vi "Write.vi"(8 "error in (no error)":errorcluster, 10 "Boolean":bool, 11 "Boolean Constant in":refnum<class "Boolean.lvclass">) -> (0 "error out":errorcluster, 3 "Boolean Constant out":refnum<class "Boolean.lvclass">)   [LabVIEW 2021, in "Variable.lvlib" / "Boolean.lvclass"]
uses:
  Boolean.lvclass
  Boolean.lvclass/Boolean.ctl
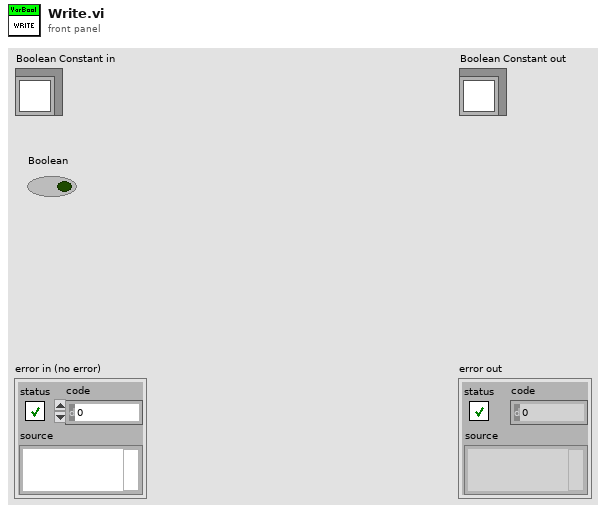
[diagram p1: front panel]
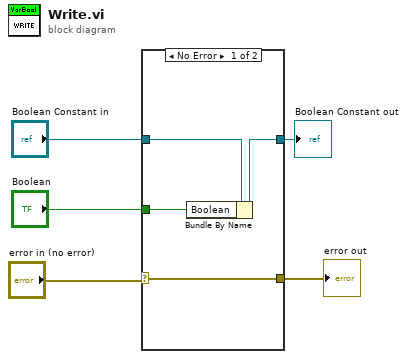
[diagram p0: block diagram]
diagram:
  n1 = case shown="No Error" "error in (no error)" {
    selector: "error in (no error)" -> [w6 w10]
    tunnel: "Boolean Constant in" -> [w9 w11]
    tunnel: [w8 w11] -> w4
    tunnel: "Boolean" -> [w7 _]
    tunnel: [w6 w10] -> w1
    frame No Error {
      n2 = Bundle By Name(cluster=w9, "Boolean"=w7) -> (w8:refnum<class "Boolean.lvclass">)
    }
    frame Error {
    }
  }
  "error out" <- w1
  "Boolean Constant out" <- w4
